vi "SetTo0.vi"(10 "Longueur d'onde":dbl) -> (2 "Température 0":dbl)   [LabVIEW 2022 SP3]
uses:
  <vilib>/DAQmx/read.llb/DAQmx Read (Analog 1D Wfm NChan NSamp).vi
  <vilib>/Analysis/baseanly.llb/Mean (DBL).vi
  <vilib>/DAQmx/create/channels.llb/DAQmx Create Channel (AI-Voltage-Basic).vi
  <vilib>/DAQmx/configure/timing.llb/DAQmx Timing (Sample Clock).vi
  <vilib>/DAQmx/miscellaneous.llb/DAQmx Fill In Error Info.vi
  <vilib>/Analysis/NI_AALBase.lvlib
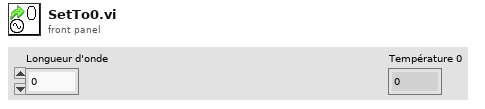
[diagram p1: front panel]
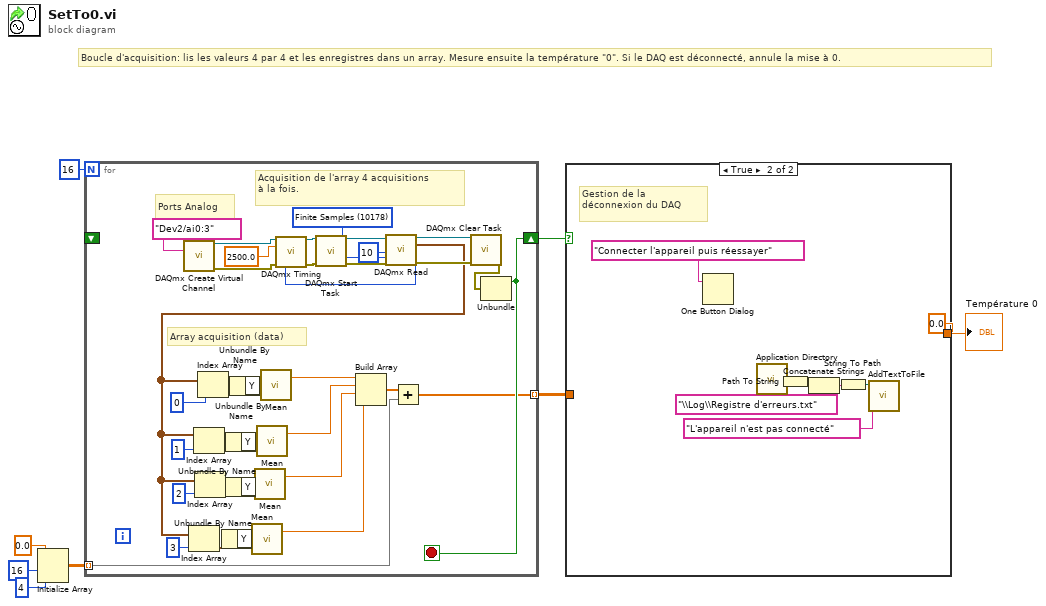
[diagram p0: block diagram]
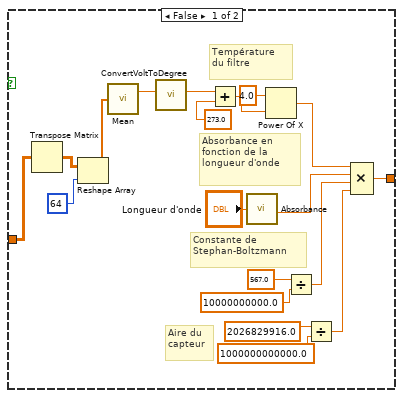
[diagram p2: hidden frame]
diagram:
  # "Boucle d'acquisition: lis les valeurs 4 par 4 et les enregistres dans un array. Mesure ensuite la température \"0\". Si le DAQ est déconnecté, annule la mise à 0."
  n1 = Initialize Array(0.0 ("element"), 16 ("dimension size"), 4 ("dimension size")) -> (w3:dbl[][])
  n2 = for {
    N: 16 -> [_]
    shift-right: [w16] -> w7
    shift-left: _ -> [_]
    tunnel: w3 -> [w10] mode=indexing
    tunnel: [w9] -> w1 mode=indexing
    stop <- w16 stop-if-true
    w20 = 10178 items=["Finite Samples"=10178, "Continuous Samples"=10123, "Hardware Timed Single Point"=12522] ("sample mode")
    # "Ports Analog"
    # "Array acquisition (data)"
    # "Acquisition de l'array 4 acquisitions\nà la fois."
    n3 = call-poly <vilib>:"DAQmx Create Virtual Channel.vi"("physical channels"=tag "Dev2/ai0:3") -> ("task out"=w41:refnum<k21>, "error out"=w40:errorcluster)  [unwired: 13 in]
    n4 = call-poly <vilib>:"DAQmx Timing.vi"("task/channels in"=w41, "sample mode"=w20, "rate"=2500.0, "error in"=w40) -> ("task out"=w37:refnum<k21>, "error out"=w38:errorcluster)  [unwired: 10 in]
    n5 = call <vilib>:"DAQmx Start Task.vi"("task/channels in"=w37, "error in"=w38) -> ("task out"=w39:refnum<k21>, "error out"=w42:errorcluster)  [unwired: 12 in]
    n6 = call-poly <vilib>:"DAQmx Read.vi"("task/channels in"=w39, "number of samples per channel"=10, "error in"=w42) -> ("task out"=w27:refnum<k21>, "data"=w17:waveform(dbl)[], "error out"=w26:errorcluster)  [unwired: 10 in]
    n7 = Index Array(array=w17, index=3) -> (element=w32:waveform(dbl))
    n8 = Index Array(array=w17, index=1) -> (element=w34:waveform(dbl))
    n9 = Index Array(array=w17, index=2) -> (element=w33:waveform(dbl))
    n10 = Index Array(array=w17, index=0) -> (element=w35:waveform(dbl))
    n11 = Unbundle By Name(w32) -> ("Y"=w28:dbl[])
    n12 = Unbundle By Name(w34) -> ("Y"=w30:dbl[])
    n13 = Unbundle By Name(w33) -> ("Y"=w29:dbl[])
    n14 = Unbundle By Name(w35) -> ("Y"=w31:dbl[])
    n15 = call-poly <vilib>:"Mean.vi"("X"=w28) -> ("mean"=w12:dbl)  [unwired: 1 out]
    n16 = call-poly <vilib>:"Mean.vi"("X"=w29) -> ("mean"=w13:dbl)  [unwired: 1 out]
    n17 = call-poly <vilib>:"Mean.vi"("X"=w30) -> ("mean"=w14:dbl)  [unwired: 1 out]
    n18 = call-poly <vilib>:"Mean.vi"("X"=w31) -> ("mean"=w15:dbl)  [unwired: 1 out]
    n19 = Build Array(w15, w14, w13, w12) -> (w11:dbl[])
    n20 = Add(x=w11, y=w10) -> (x+y=w9:dbl[])
    n21 = call <vilib>:"DAQmx Clear Task.vi"("task in"=w27, "error in"=w26) -> ("error out"=w36:errorcluster)  [unwired: 13 in]
    n22 = Unbundle(w36) -> ("status"=w16:bool)  [unwired: 2 out]
  }
  n23 = case shown="True" w7 {
    tunnel: w1 -> [w47 _]
    tunnel: [w43 0.0] -> w2
    frame False {
      # "Constante de \nStephan-Boltzmann"
      # "Absorbance en\nfonction de la \nlongueur d'onde"
      # "Température \ndu filtre"
      # "Aire du\ncapteur"
      n24 = Transpose Matrix(1:w47) -> (0:w48:dbl[][])
      n25 = Reshape Array(w48, 64 ("dimension size")) -> (w45:dbl[])
      n26 = call-poly <vilib>:"Mean.vi"("X"=w45) -> ("mean"=w44:dbl)  [unwired: 1 out]
      n27 = call "ConvertVoltToDegree.vi"("Tension"=w44) -> ("Température"=w53:dbl)  [unwired: 10 in]
      n28 = Add(x=w53, y=273.0) -> (x+y=w60:dbl)
      n29 = call "Absorbance.vi"("Longueur d'onde"="Longueur d'onde") -> ("absorbance"=w50:dbl)  [unwired: 10 in]
      n30 = Power Of X(1:w60, 2:4.0 ("y")) -> (0:w49:dbl)
      n31 = Divide(x=567.0, y=10000000000.0) -> (x/y=w51:dbl)
      n32 = Divide(x=2026829916.0, y=1000000000000.0) -> (x/y=w52:dbl)
      n33 = Compound Arithmetic op=MULTIPLY(w49, w50, w51, w52) -> (w43:dbl)
    }
    frame True {
      # "Gestion de la \ndéconnexion du DAQ"
      n34 = One Button Dialog(message="Connecter l'appareil puis réessayer") -> ()  [unwired: 1 in, 1 out]
      n35 = call <vilib>:"Application Directory.vi"() -> ("Application Directory"=w65:path)
      n36 = Path To String(path=w65) -> (string=w66:string)
      n37 = Concatenate Strings(w66, "\\Log\\Registre d'erreurs.txt") -> (w67:string)
      n38 = String To Path(string=w67) -> (path=w63:path)
      n39 = call "AddTextToFile.vi"("Ajouter du texte"="L'appareil n'est pas connecté", "Fichier"=w63) -> ()  [unwired: 10 in]
    }
  }
  "Température 0" <- w2
